vi "GetSinglePointChannelProperties.vi"(11 "channel":T2) -> (2 "TDMS properties":T1[](array[typedef]))   [LabVIEW 2017, in "Tdms.lvlib"]
doc: "Returns TDMS properties that define how a single-point channel works. Use the TDMS Set Properties function to write these properties to a TDMS file that contains data from the channel."
uses:
  <vilib>/addons/InsightCM/Utilities/Tdms/Tdms.lvlib
  <vilib>/addons/InsightCM/MessageBus/Base/controls/R2_Channel.ctl
  <vilib>/addons/InsightCM/MessageBus/Base/controls/KeyValuePair.ctl
  <vilib>/addons/InsightCM/MessageBus/Base/controls/Metric.ctl
  <vilib>/addons/InsightCM/Utilities/Tdms/controls/Property.ctl
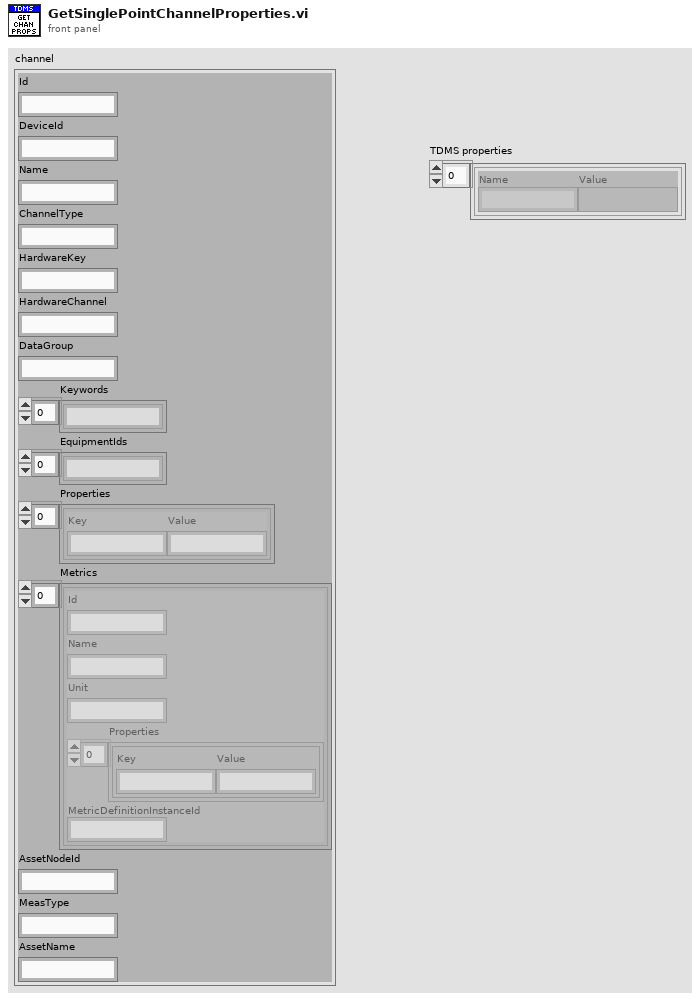
[diagram p1: front panel]
types:
  T1 = typedef "Tdms.lvlib/Property.ctl" = cluster{"Name":string, "Value":variant}
  T2 = typedef "R2_Channel.ctl" = cluster{"Id":string, "DeviceId":string, "Name":string, "ChannelType":string, "HardwareKey":string, "HardwareChannel":string, "DataGroup":string, "Keywords":string[], "EquipmentIds":string[], "Properties":T3[], "Metrics":T4[], "AssetNodeId":string, "MeasType":string, "AssetName":string}
  T3 = typedef "KeyValuePair.ctl" = cluster{"Key":string, "Value":string}
  T4 = typedef "Metric.ctl" = cluster{"Id":string, "Name":string, "Unit":string, "Properties":T3[], "MetricDefinitionInstanceId":string}
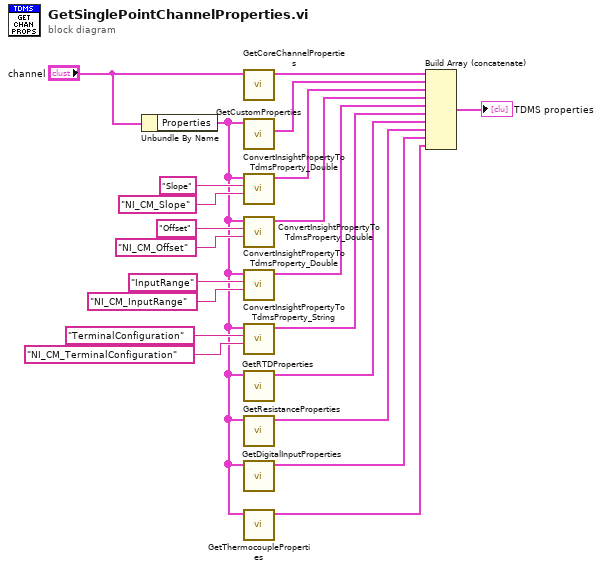
[diagram p0: block diagram]
diagram:
  n1 = Unbundle By Name("channel") -> ("Properties"=w6:T3[])
  n2 = call <vilib>:"GetCoreChannelProperties.vi"("Channel"="channel") -> ("Tdms Properties"=w20:T1[])  [unwired: 10 in]
  n3 = call <vilib>:"GetCustomProperties.vi"("Properties"=w6) -> ("Tdms Properties"=w19:T1[])  [unwired: 10 in]
  n4 = call <vilib>:"ConvertInsightPropertyToTdmsProperty_Double.vi"("Tdms Property Name"="NI_CM_Slope" ("Name"), "Insight Property Name"="Slope" ("Name"), "Insight Properties"=w6) -> ("Tdms Properties"=w13:T1[])  [unwired: 8 in]
  n5 = call <vilib>:"ConvertInsightPropertyToTdmsProperty_Double.vi"("Tdms Property Name"="NI_CM_Offset" ("Name"), "Insight Property Name"="Offset" ("Name"), "Insight Properties"=w6) -> ("Tdms Properties"=w12:T1[])  [unwired: 8 in]
  n6 = call <vilib>:"ConvertInsightPropertyToTdmsProperty_Double.vi"("Tdms Property Name"="NI_CM_InputRange" ("Name"), "Insight Property Name"="InputRange" ("Name"), "Insight Properties"=w6) -> ("Tdms Properties"=w9:T1[])  [unwired: 8 in]
  n7 = call <vilib>:"ConvertInsightPropertyToTdmsProperty_String.vi"("Tdms Property Name"="NI_CM_TerminalConfiguration" ("Name"), "Insight Property Name"="TerminalConfiguration" ("Name"), "Insight Properties"=w6) -> ("Tdms Properties"=w5:T1[])  [unwired: 8 in]
  n8 = call <vilib>:"GetRTDProperties.vi"("channel properties"=w6) -> ("tdms properties"=w4:T1[])  [unwired: 10 in]
  n9 = call <vilib>:"GetResistanceProperties.vi"("channel properties"=w6) -> ("tdms properties"=w3:T1[])  [unwired: 10 in]
  n10 = call <vilib>:"GetDigitalInputProperties.vi"("channel properties"=w6) -> ("tdms properties"=w2:T1[])  [unwired: 10 in]
  n11 = call <vilib>:"GetThermocoupleProperties.vi"("channel properties"=w6) -> ("tdms properties"=w1:T1[])  [unwired: 10 in]
  n12 = Build Array (concatenate)(w20, w19, w13, w12, w9, w5, w4, w3, w2, w1) -> (→"TDMS properties":T1[])
